vi "Get Coverage Percentage.vi"(8 "error in (no error)":errorcluster, 10 "VI Path":path, 11 "CodeCoverage in":refnum<class "Code Coverage.lvclass">) -> (0 "error out":errorcluster, 2 "Coverage Percentage":dbl, 3 "CodeCoverage out":refnum<class "Code Coverage.lvclass">)   [LabVIEW 2017, in "Code Coverage.lvclass"]
doc: "Returns the code coverage percentage for a given VI."
uses:
  Code Coverage.lvclass
  Code Coverage.lvclass/Code Coverage.ctl
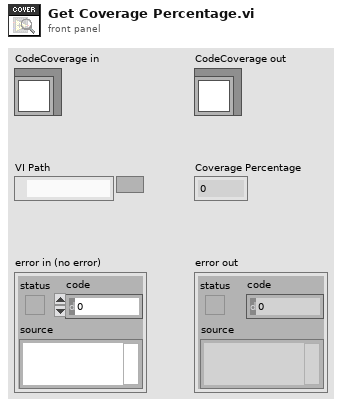
[diagram p1: front panel]
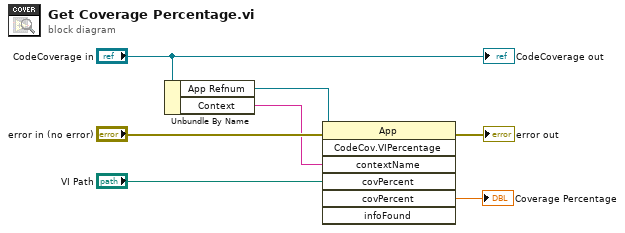
[diagram p0: block diagram]
diagram:
  n1 = Unbundle By Name("CodeCoverage in") -> ("App Refnum"=w3:refnum<vi>, "Context"=w2:string)
  n2 = invoke class="App" method="CodeCov.VIPercentage"(reference=w3, error in="error in (no error)", "contextName"=w2, "covPercent"="VI Path") -> (error out=→"error out":errorcluster, "covPercent"=→"Coverage Percentage":dbl)  [unwired: 3 in, 5 out]
  "CodeCoverage out" <- "CodeCoverage in"
